vi "Varint Base128 Decoder.vi"(11 "Array":u8[](array[numeric]) format="%02x") -> (2 "array w/ subset deleted":u8[](array[numeric]), 3 "Numeric":i32)   [LabVIEW 2017]
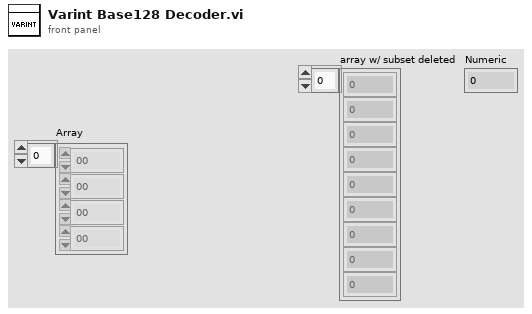
[diagram p1: front panel]
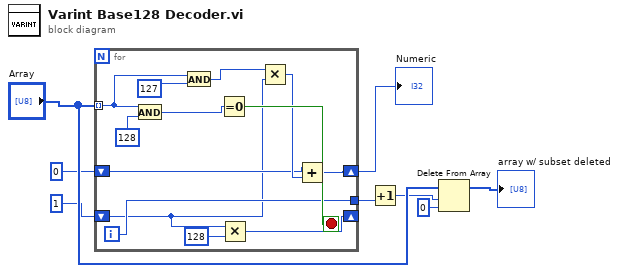
[diagram p0: block diagram]
diagram:
  n1 = for {
    tunnel: "Array" -> [w17] mode=indexing
    tunnel: [w18] -> w5
    shift-right: [w12] -> w1
    shift-left: 0 -> [w13]
    shift-right: [w10] -> _
    shift-left: 1 -> [w11]
    i -> [w18]
    stop <- w19 stop-if-true
    n2 = And(x=w17, y=u8 128 ("x")) -> (x .and. y?=w20:u8)
    n3 = And(x=w17, y=u8 127) -> (x .and. y?=w15:u8)
    n4 = Equal To 0?(x=w20) -> (x = 0?=w19:bool)
    n5 = Multiply(x=w11, y=128) -> (x*y=w10:i32)
    n6 = Multiply(x=w15, y=w11) -> (x*y=w14:i32)
    n7 = Add(x=w13, y=w14) -> (x+y=w12:i32)
  }
  "Numeric" <- w1
  n8 = Increment(x=w5) -> (x+1=w4:i32)
  n9 = Delete From Array(array="Array", length=w4, index=0) -> (array with subset deleted=→"array w/ subset deleted":u8[])  [unwired: 1 out]
